vi "Write Wrapback Data.vi"(0 "I data":fxp<+/-,16,1>[](array[numeric])=[0.0, 0.0, 0.0, 0.0, 0.0, 0.0, 0.0, 0.0, 0.0, 0.0, 0.0, 0.0, 0.0, 0.0, 0.0, 0.0], 2 "shared":refnum<class "niUSRP Rx Core v1 FPGA.lvclass">=refnum, 5 "Q data":fxp<+/-,16,1>[](array[numeric])=[0.0, 0.0, 0.0, 0.0, 0.0, 0.0, 0.0, 0.0, 0.0, 0.0, 0.0, 0.0, 0.0, 0.0, 0.0, 0.0]) -> ()   [LabVIEW 2023, in "niUSRP Rx Core v1 FPGA.lvclass"]
doc: "this VI is used to wrap data from Generation output to Acquisition input."
uses:
  <instrlib>/niUSRP/Reference FPGA/Rx Core/niUSRP Rx Core v1 FPGA.lvclass
  <vilib>/rvi/DataTransferAndStorage/Container/XNode/niFpgaContainer.xnode
  <vilib>/rvi/DataTransferAndStorage/Register/Emulation/niFpgaRegisterEmulationRefIn.vi
  <instrlib>/niVST/Reference FPGA/FPGA/niUSRP Rx Core v1 FPGA/niUSRP Rx Core v1 FPGA.lvclass
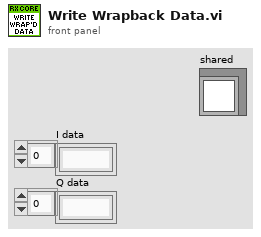
[diagram p1: front panel]
types:
  T1 = cluster{"I data":fxp<+/-,16,1>[], "Q data":fxp<+/-,16,1>[]}
  T2 = typedef "niVST Shared Registers v1 FPGA.lvclass/Shared Registers.ctl" = cluster{"wrapback data":refnum<k21>, "status.gen.generating":refnum<k21>, "status.gen.waiting for trigger":refnum<k21>, "status.acq.in progress":refnum<k21>, "status.acq.waiting for trigger":refnum<k21>}
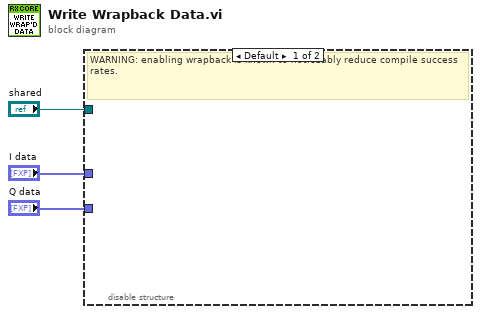
[diagram p0: block diagram]
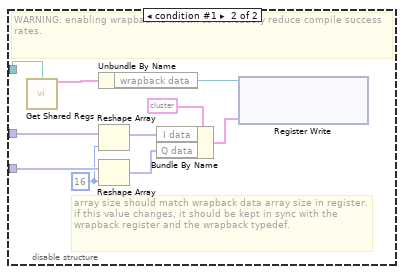
[diagram p2: hidden frame]
diagram:
  n1 = disable-structure shown="Default" {
    disable-tunnel: "shared" -> [_ w4]
    disable-tunnel: "I data" -> [_ w10]
    disable-tunnel: "Q data" -> [_ w9]
    frame condition #0 (active) {
      # "WARNING: enabling wrapback is known to noticeably reduce compile success rates."
    }
    frame condition #1 {
      w6 = 16 ("dimension size")
      # "array size should match wrapback data array size in register. if this value changes, it should be kept in sync with the wrapback register and the wrapback typedef."
      # "WARNING: enabling wrapback is known to noticeably reduce compile success rates."
      n2 = call-dynamic "Get Shared Regs.vi"("shared"=w4) -> ("shared regs"=w5:T2)  [unwired: 14 in]
      n3 = Unbundle By Name(w5) -> ("wrapback data"=w13:refnum<k21>)
      n4 = Reshape Array(w10, w6) -> (w8:fxp<+/-,16,1>[])
      n5 = Reshape Array(w9, w6) -> (w7:fxp<+/-,16,1>[])
      n6 = Bundle By Name(cluster=T1 {"I data"=[0.0, 0.0, 0.0, 0.0, 0.0, 0.0, 0.0, 0.0, 0.0, 0.0, 0.0, 0.0, 0.0, 0.0, 0.0, 0.0], "Q data"=[0.0, 0.0, 0.0, 0.0, 0.0, 0.0, 0.0, 0.0, 0.0, 0.0, 0.0, 0.0, 0.0, 0.0, 0.0, 0.0]} ("Data"), "I data"=w8, "Q data"=w7) -> (w11:T1)
      n7 = xnode "Register Write"("Data"=w11, "Register In"=w13) -> ()  [unwired: 1 out]
    }
  }
